vi "Scaling (Ratio).vi"(0 "waveforms in":waveform(dbl)[](array[waveform]), 5 "CT/VT ratio":cluster{"primary":dbl, "secondary":dbl}[](array[cluster]), 9 "system info in":refnum<class "EP System Info.lvclass">, 11 "error in (no error)":errorcluster) -> (4 "waveforms out":waveform(dbl)[](array[waveform]), 10 "system info out":refnum<class "EP System Info.lvclass">, 15 "error out":errorcluster)   [LabVIEW 2014, in "NI_EP_Power Quality.lvlib"]
doc: "Scales waveforms based on the sensitivity of the voltage/current transformer or transducer. You must manually select the polymorphic instance you want to use.\n\nThis VI supports measuring single-line and multiple-line systems."
uses:
  <vilib>/addons/Electrical Power/PQ/NI_EP_Power Quality.lvlib
  <vilib>/addons/Electrical Power/PQ/Common/Classes/System Info/EP System Info.lvclass
panel:
  # ":"
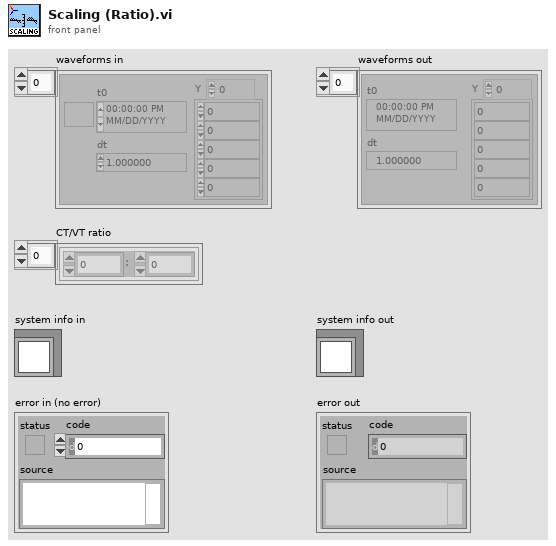
[diagram p1: front panel]
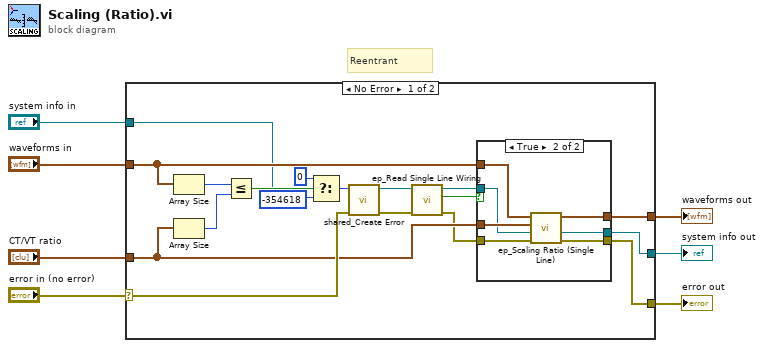
[diagram p0: block diagram]
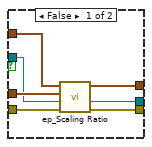
[diagram p2: hidden frame]
diagram:
  # "Reentrant"
  n1 = case shown="No Error" "error in (no error)" {
    selector: "error in (no error)" -> [w18 w41]
    tunnel: "waveforms in" -> [w17 w40]
    tunnel: "CT/VT ratio" -> [w16 _]
    tunnel: "system info in" -> [w15 w39]
    tunnel: [w13 w41] -> w4
    tunnel: [w14 w39] -> w3
    tunnel: [w12 w40] -> w2
    frame No Error {
      n2 = Array Size(array=w17) -> (size(s)=w23:i32)
      n3 = Array Size(array=w16) -> (size(s)=w24:i32)
      n4 = Less Or Equal?(x=w23, y=w24) -> (x <= y?=w22:bool)
      n5 = Select(t=0 ("error code (0)"), s=w22, f=-354618 ("error code (0)")) -> (s? t:f=w19:i32)
      n6 = call <vilib>:"shared_Create Error.vi"("error in (no error)"=w18, "error code (0)"=w19) -> ("error out"=w9:errorcluster)  [unwired: 9 in]
      n7 = call <vilib>:"ep_Read Single Line Wiring.vi"("error in (no error)"=w9, "system info in"=w15) -> ("error out"=w8:errorcluster, "single line wiring? (F)"=w10:bool, "system info out"=w11:refnum<class "EP System Info.lvclass">)  [unwired: 7 in]
      n8 = case shown="True" w10 {
        tunnel: w17 -> [w31 w38]
        tunnel: w16 -> [w30 w37]
        tunnel: [w26 w36] -> w14
        tunnel: w8 -> [w28 w35]
        tunnel: [w27 w34] -> w13
        tunnel: [w25 w33] -> w12
        tunnel: w11 -> [w29 w32]
        frame False {
          n9 = call <vilib>:"ep_Scaling Ratio.vi"("error in (no error)"=w28, "system info in"=w29, "CT/VT ratio"=w30, "waveforms in"=w31) -> ("error out"=w27:errorcluster, "system info out"=w26:refnum<class "EP System Info.lvclass">, "waveforms out"=w25:waveform(dbl)[])  [unwired: 5 in]
        }
        frame True {
          n10 = call <vilib>:"ep_Scaling Ratio (Single Line).vi"("error in (no error)"=w35, "system info in"=w32, "CT/VT ratio"=w37, "waveforms in"=w38) -> ("error out"=w34:errorcluster, "system info out"=w36:refnum<class "EP System Info.lvclass">, "waveforms out"=w33:waveform(dbl)[])  [unwired: 5 in]
        }
      }
    }
    frame Error {
    }
  }
  "waveforms out" <- w2
  "error out" <- w4
  "system info out" <- w3
